vi "Main.vi"() -> ()   [LabVIEW 2013]
uses:
  Type Definitions/3D Model Status.ctl
  Bluetooth/Bluetooth status.ctl
  Type Definitions/Settings File Name.ctl
  <vilib>/Utility/miscctls.llb/LV3DPointTypeDef.ctl
  <vilib>/Instr/_visa.llb/VISA Flush IO Buffer Mask.ctl
  <vilib>/Instr/_visa.llb/VISA Set IO Buffer Mask.ctl
  <vilib>/Utility/xml.llb/Read From XML File(string).vi
  <vilib>/Utility/xml.llb/Write to XML File(string).vi
  <vilib>/picture/3D Picture Control/Object/Create Object (name).vi
  <vilib>/Instr/_visa.llb/VISA Configure Serial Port (Instr).vi
  <vilib>/picture/3D Picture Control/NI_3D Picture Control.lvlib
panel:
  out "Acquire [ms]":u32
  out "Sending [ms]":u32
  in  "VISA resource name":refnum<visa-resource-name>
  in  "Motor 4":u8(slide) scale=0.0..100.0
  in  "Motor 3":u8(slide) scale=0.0..100.0
  in  "Motor 2":u8(slide) scale=0.0..100.0
  in  "Motor 1":u8(slide) scale=0.0..100.0
  out "Press Low":i32 caption="X"
  out "Press High":i32 caption="X"
  out "Temperature":i32
  out "Z Axis":sgl
  out "Zyro 1":i32 caption="X"
  out "Zyro 2":i32 caption="X"
  out "Zyro 3":i32 caption="X"
  out "Zyro 4":i32 caption="X"
  out "Y_Low":i32 caption="Y"
  out "X_Low":i32 caption="X"
  out "Y Axis":sgl
  out "X Axis":sgl
  in  "Stop Bluetooth Button":bool
  in  "Bluetooth Connect Button":bool
  out "Battery":i32
  out "Y_High":i32 caption="Y"
  out "X_High":i32 caption="X"
  out "3D Picture":refnum<vi>(3d-picture)
  in  "Load Model":bool
  in  "Stop Button":bool
  in  "Path to STL File":path=path "C:/Users/Marcin/SkyDrive/Dokumenty/Quadrocopter/LabVIEW 3D Model/Zlozenie.stl"
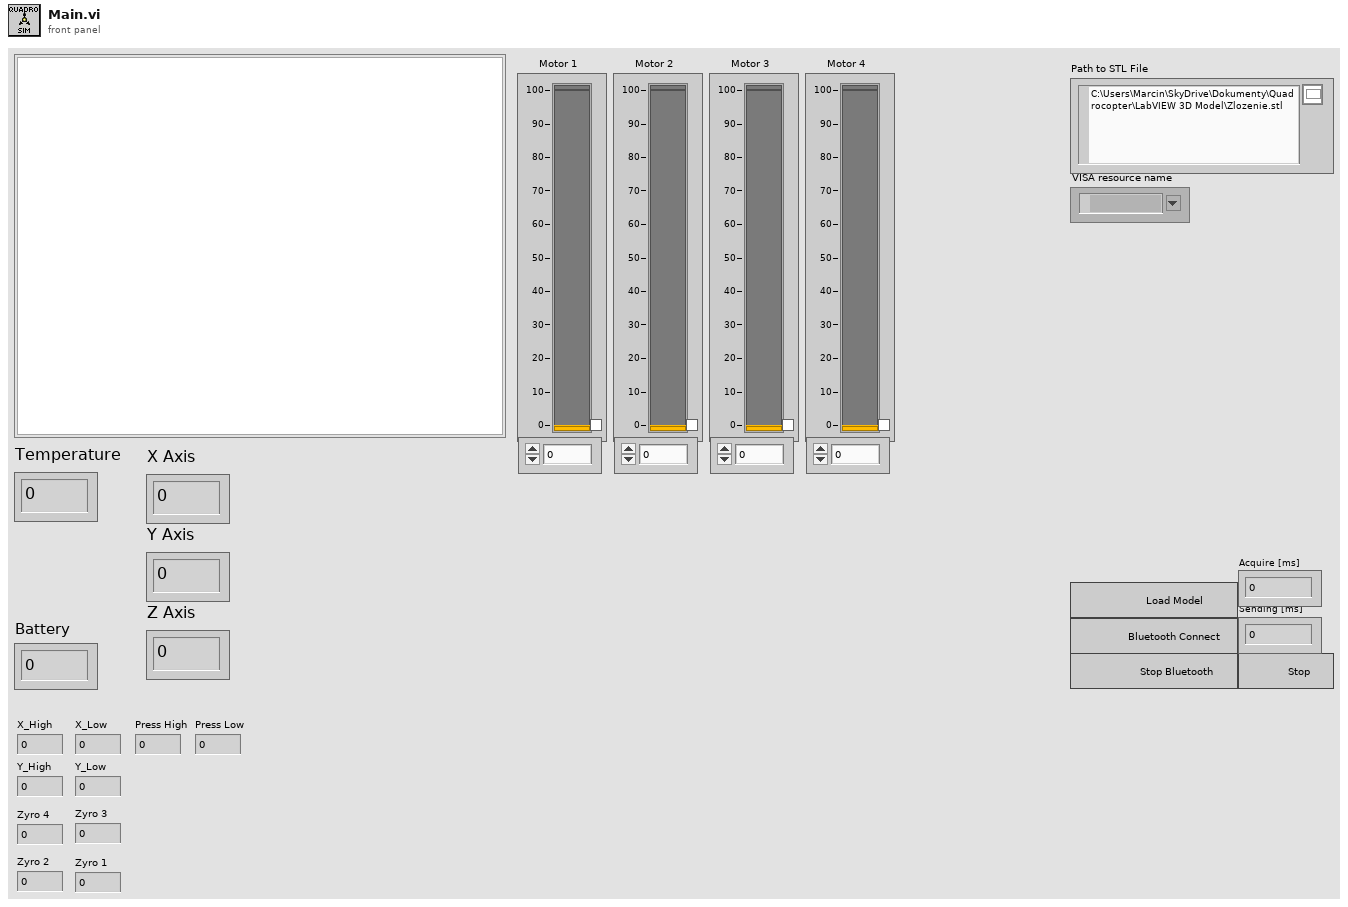
[diagram p1: front panel]
types:
  T1 = typedef "Bluetooth status.ctl" = enum16{"Idle", "Connected"}
  T2 = typedef "3D Model Status.ctl" = enum16{"Idle", "Update"}
  T3 = typedef "VISA Set IO Buffer Mask.ctl" = u16
  T4 = typedef "VISA Flush IO Buffer Mask.ctl" = u16
  T5 = typedef "Settings File Name.ctl" = string
  T6 = typedef "LV3DPointTypeDef.ctl" = cluster{"X":sgl, "Y":sgl, "Z":sgl}
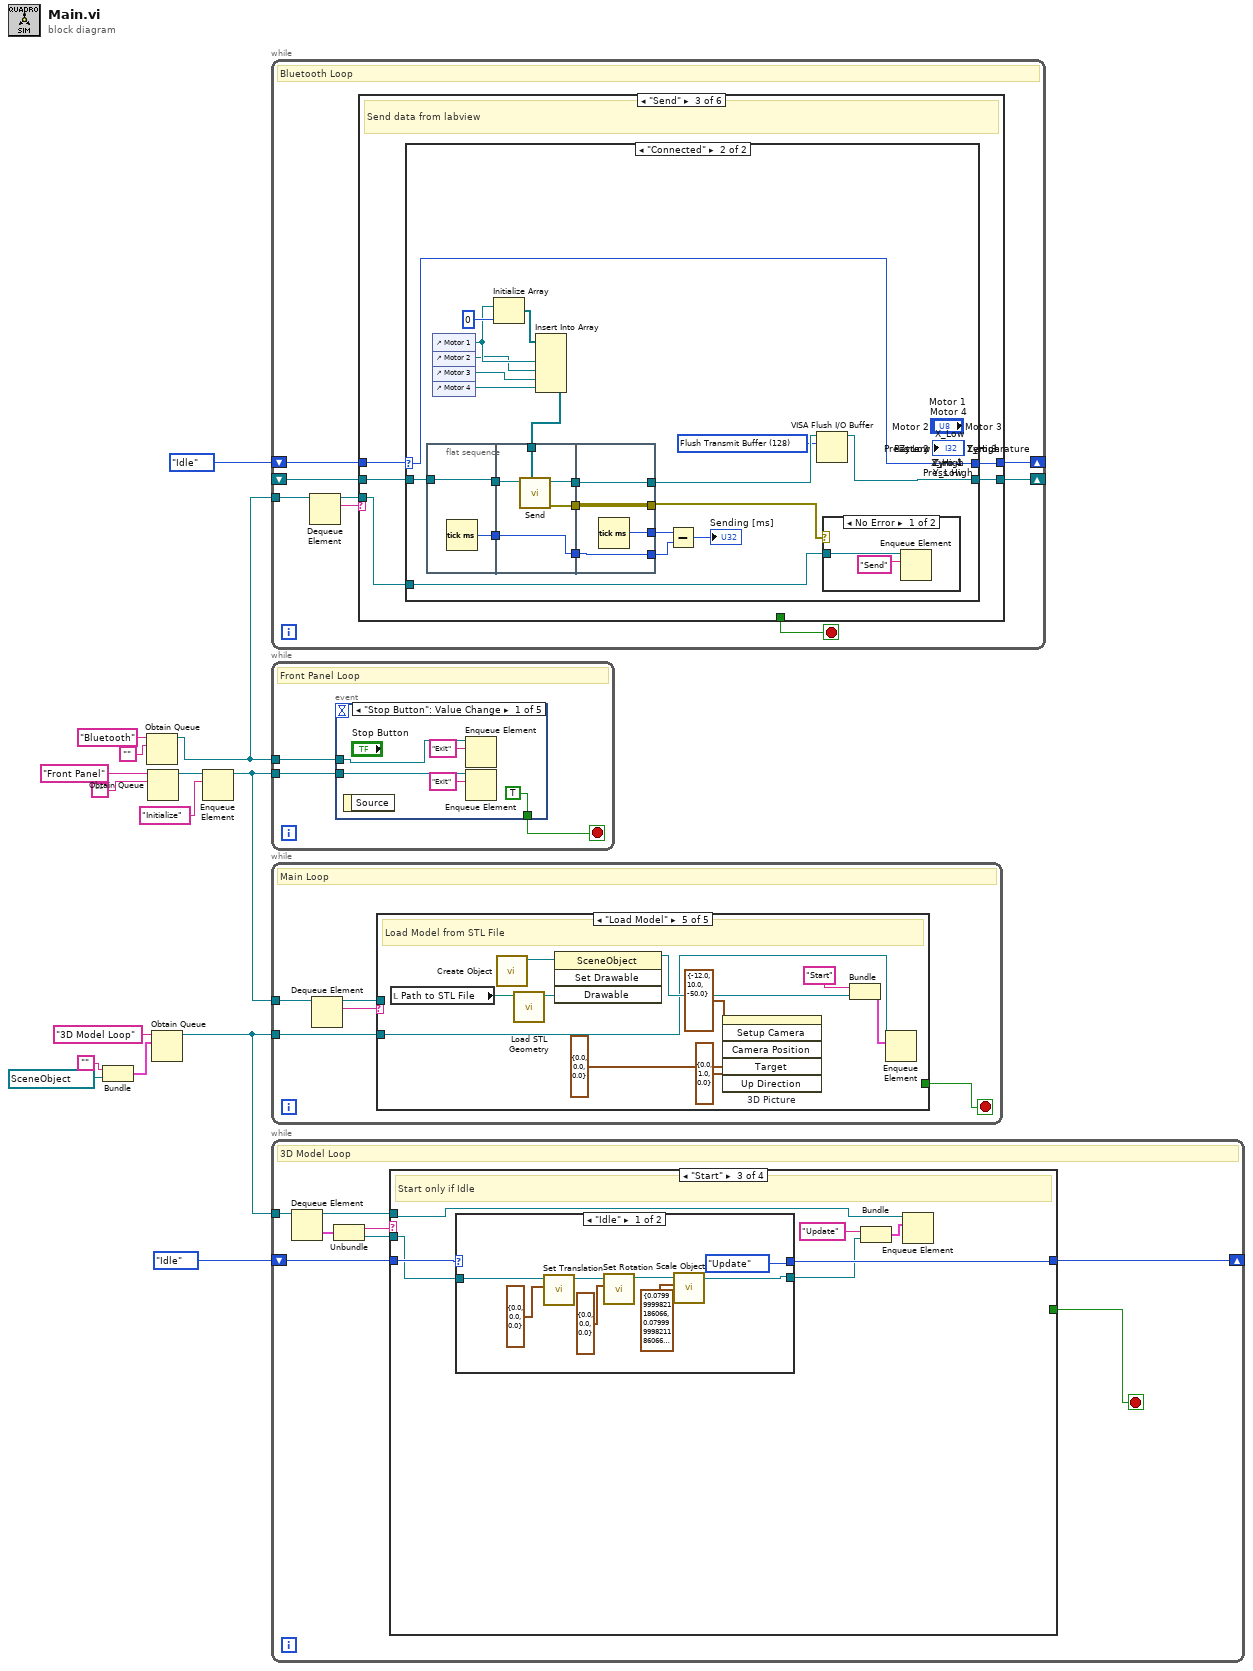
[diagram p0: block diagram]
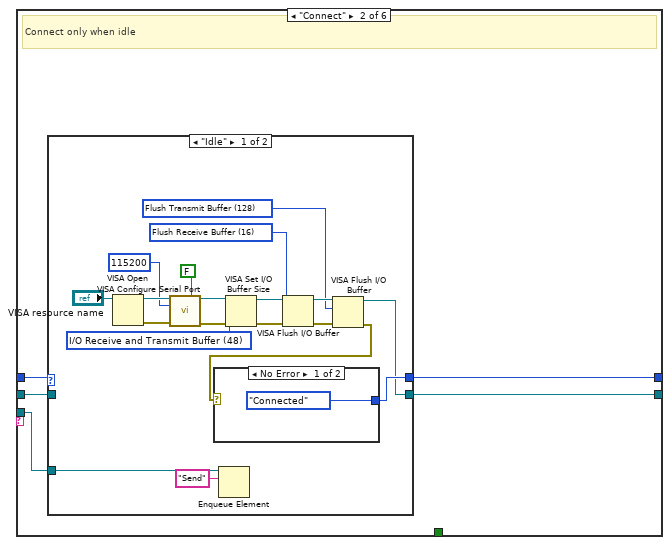
[diagram p3: hidden frame]
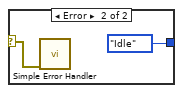
[diagram p4: hidden frame]
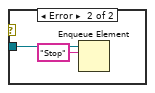
[diagram p7: hidden frame]
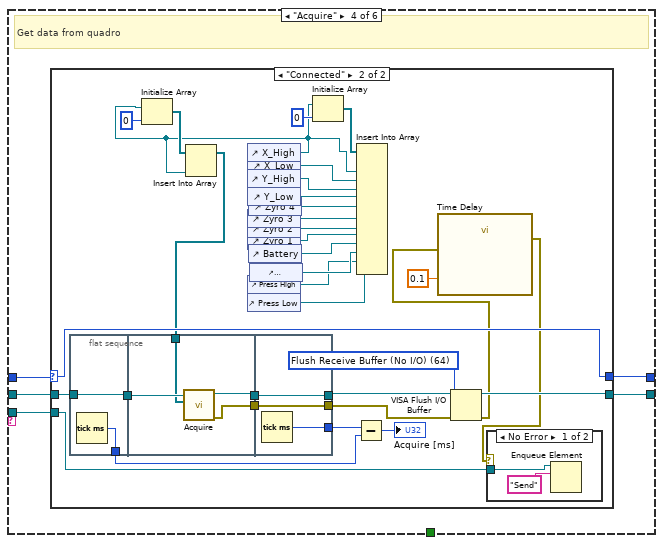
[diagram p8: hidden frame]
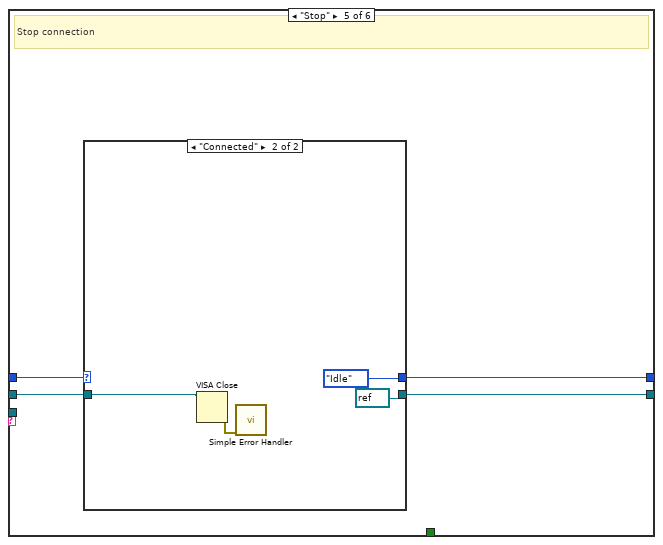
[diagram p11: hidden frame]
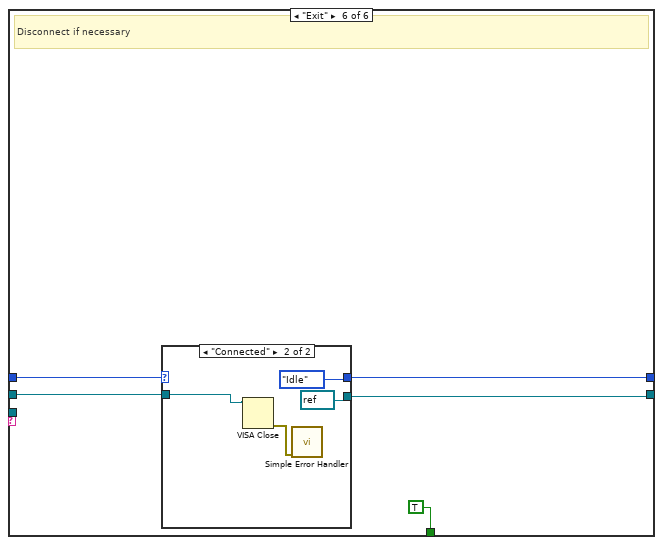
[diagram p13: hidden frame]
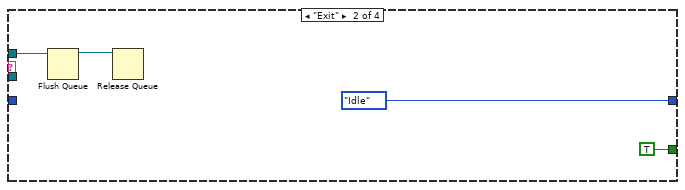
[diagram p16: hidden frame]
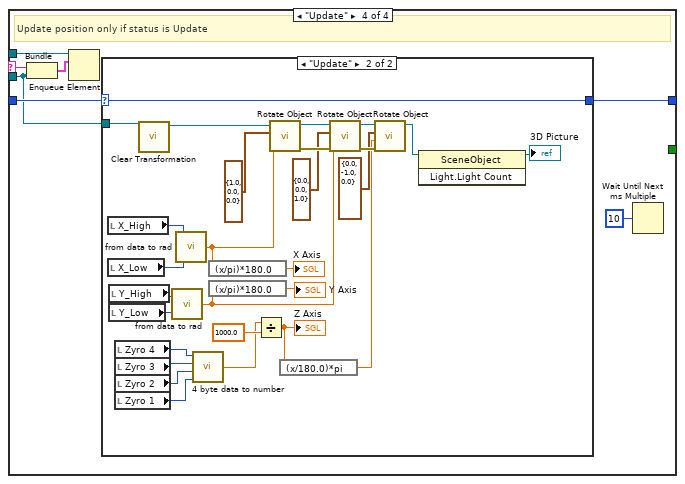
[diagram p18: hidden frame]
diagram:
  n1 = Bundle("", "reference out"=refnum<vi> refnum) -> (w5:cluster{string, "reference out":refnum<vi>})  [unwired: 1 in]
  n2 = Obtain Queue(name (unnamed)="Bluetooth", element data type="") -> (queue out=w2:refnum<queue>)  [unwired: 3 in, 2 out]
  n3 = Obtain Queue(name (unnamed)="Front Panel", element data type="") -> (queue out=w13:refnum<queue>)  [unwired: 3 in, 2 out]
  n4 = Obtain Queue(name (unnamed)="3D Model Loop", element data type=w5) -> (queue out=w9:refnum<queue>)  [unwired: 3 in, 2 out]
  n5 = Enqueue Element(queue=w13, element="Initialize") -> (queue out=w11:refnum<queue>)  [unwired: 2 in, 2 out]
  n6 = while {
    tunnel: w2 -> [w22]
    shift-right: [w19] -> _
    shift-left: Bluetooth_status."Idle" -> [w20]
    shift-right: [w18] -> _
    shift-left: _ -> [w17]
    stop <- w16 stop-if-true
    # "Bluetooth Loop"
    n7 = Dequeue Element(queue=w22) -> (queue out=w21:refnum<queue>, element=w23:string)  [unwired: 2 in, 2 out]
    n8 = case shown="\"Send\"" w23 {
      tunnel: w21 -> [_ w26 w55 w99 _ _]
      tunnel: w20 -> [w24 w30 w59 w103 w153 w163]
      tunnel: [w24 w29 w58 w102 w151 w160] -> w19
      tunnel: [w25 w28 w57 w100 w150 w161] -> w18
      tunnel: w17 -> [w25 w27 w56 w101 w152 w162]
      tunnel: [_ _ _ _ _ TRUE] -> w16
      frame Default {
        # "Do nothing"
      }
      frame "Connect" {
        # "Connect only when idle"
        n9 = case shown="\"Idle\"" w30 {
          selector: w30 -> [_ w53]
          tunnel: [w47 w53] -> w29
          tunnel: [w33 w54] -> w28
          tunnel: w27 -> [_ w54]
          tunnel: w26 -> [w49 _]
          frame "Idle" {
            w31 = T3 48 items=["I/O Receive Buffer"=16, "I/O Transmit Buffer"=32, "I/O Receive and Transmit Buffer"=48] ("Mask")
            w32 = T4 128 items=["Flush Receive Buffer"=16, "Write Transmit Buffer to Device"=32, "Flush Receive Buffer (No I/O)"=64, "Flush Transmit Buffer"=128] ("Mask")
            w37 = T4 16 items=["Flush Receive Buffer"=16, "Write Transmit Buffer to Device"=32, "Flush Receive Buffer (No I/O)"=64, "Flush Transmit Buffer"=128] ("Mask")
            n10 = VISA Open(VISA resource name="VISA resource name") -> (VISA resource name=w46:refnum<visa-resource-name>, error out=w45:errorcluster)  [unwired: 4 in]
            n11 = call-poly "VISA Configure Serial Port"("VISA resource name"=w46, "Enable Termination\nChar (T)"=FALSE ("Enable Termination\nChar (T)"), "baud rate (9600)"=u32 115200, "error in (no error)"=w45) -> ("VISA resource name out"=w43:refnum<visa-resource-name>, "error out"=w44:errorcluster)  [unwired: 10 in]
            n12 = Enqueue Element(queue=w49, element="Send") -> ()  [unwired: 2 in, 3 out]
            n13 = VISA Set I/O Buffer Size(VISA resource name=w43, mask (16)=w31, error in (no error)=w44) -> (VISA resource name out=w41:refnum<visa-resource-name>, error out=w42:errorcluster)  [unwired: 1 in]
            n14 = VISA Flush I/O Buffer(VISA resource name=w41, mask (16)=w37, error in (no error)=w42) -> (VISA resource name out=w35:refnum<visa-resource-name>, error out=w36:errorcluster)
            n15 = VISA Flush I/O Buffer(VISA resource name=w35, mask (16)=w32, error in (no error)=w36) -> (VISA resource name out=w33:refnum<visa-resource-name>, error out=w34:errorcluster)
            n16 = case shown="No Error" w34 {
              selector: w34 -> [_ w52]
              tunnel: [Bluetooth_status."Connected" Bluetooth_status."Idle"] -> w47
              frame No Error {
              }
              frame Error {
                n17 = call <vilib>:"Simple Error Handler.vi"("error in (no error)"=w52) -> ()  [unwired: 4 in, 5 out]
              }
            }
          }
          frame "Connected", Default {
          }
        }
      }
      frame "Send" {
        # "Send data from labview"
        n18 = case shown="\"Connected\"" w59 {
          selector: w59 -> [w61 w66]
          tunnel: [w61 w66] -> w58
          tunnel: [w60 w63] -> w57
          tunnel: w56 -> [w60 w76]
          tunnel: w55 -> [_ w83]
          frame "Idle", Default {
          }
          frame "Connected" {
            w62 = T4 128 items=["Flush Receive Buffer"=16, "Write Transmit Buffer to Device"=32, "Flush Receive Buffer (No I/O)"=64, "Flush Transmit Buffer"=128] ("Mask")
            n19 = flat-sequence {
              tunnel: w76 -> [w85]
              tunnel: [w85] -> w75
              tunnel: [w84] -> w69
              tunnel: w75 -> [w90]
              tunnel: w65 -> [w87]
              tunnel: [w89] -> w73
              tunnel: [w88] -> w72
              tunnel: w69 -> [w86]
              tunnel: [w86] -> w68
              tunnel: [w93] -> w74
              tunnel: [w94] -> w64
              tunnel: w73 -> [w94]
              tunnel: w72 -> [w93]
              tunnel: [w92] -> w71
              tunnel: [w91] -> w70
              tunnel: w68 -> [w91]
              frame #0 {
                n20 = Tick Count (ms)() -> (millisecond timer value=w84:u32)
              }
              frame #1 {
                n21 = call "Send.vi"("Motors input"=w87, "VISA resource name"=w90) -> ("Error Out"=w88:errorcluster, "VISA resource name out"=w89:refnum<visa-resource-name>)  [unwired: 8 in]
              }
              frame #2 {
                n22 = Tick Count (ms)() -> (millisecond timer value=w92:u32)
              }
            }
            n23 = control-ref of="Motor 1"() -> (w80:refnum<vi>)
            n24 = control-ref of="Motor 2"() -> (w79:refnum<vi>)
            n25 = control-ref of="Motor 3"() -> (w78:refnum<vi>)
            n26 = control-ref of="Motor 4"() -> (w77:refnum<vi>)
            n27 = Initialize Array(w80, 0 ("dimension size")) -> (w81:refnum<vi>[])
            n28 = Insert Into Array(array=w81, new element #1=w80, new element #2=w79, new element #3=w78, new element #4=w77) -> (w65:refnum<vi>[])  [unwired: 1 in]
            n29 = Subtract(x=w71, y=w70) -> (x-y=→"Sending [ms]":u32)
            n30 = VISA Flush I/O Buffer(VISA resource name=w64, mask (16)=w62) -> (VISA resource name out=w63:refnum<visa-resource-name>)  [unwired: 1 in, 1 out]
            n31 = case shown="No Error" w74 {
              tunnel: w83 -> [w95 w98]
              frame No Error {
                n32 = Enqueue Element(queue=w95, element="Send") -> ()  [unwired: 2 in, 3 out]
              }
              frame Error {
                n33 = Enqueue Element(queue=w98, element="Stop") -> ()  [unwired: 2 in, 3 out]
              }
            }
          }
        }
      }
      frame "Acquire" {
        # "Get data from quadro"
        n34 = case shown="\"Connected\"" w103 {
          selector: w103 -> [w105 w125]
          tunnel: [w105 w125] -> w102
          tunnel: [w104 w117] -> w100
          tunnel: w101 -> [w104 w120]
          tunnel: w99 -> [_ w115]
          frame "Idle", Default {
          }
          frame "Connected" {
            w116 = T4 64 items=["Flush Receive Buffer"=16, "Write Transmit Buffer to Device"=32, "Flush Receive Buffer (No I/O)"=64, "Flush Transmit Buffer"=128] ("Mask")
            n35 = flat-sequence {
              tunnel: [w142] -> w123
              tunnel: [w141] -> w121
              tunnel: w120 -> [w141]
              tunnel: w121 -> [w146]
              tunnel: [w145] -> w119
              tunnel: [w144] -> w114
              tunnel: w109 -> [w143]
              tunnel: [w149] -> w124
              tunnel: [w148] -> w118
              tunnel: w119 -> [w148]
              tunnel: w114 -> [w147]
              tunnel: [w147] -> w113
              frame #0 {
                n36 = Tick Count (ms)() -> (millisecond timer value=w142:u32)
              }
              frame #1 {
                n37 = call "Acquire.vi"("Controls Ref Array"=w143, "VISA resource name"=w146) -> ("error out"=w144:errorcluster, "VISA resource name out"=w145:refnum<visa-resource-name>)  [unwired: 8 in]
              }
              frame #2 {
                n38 = Tick Count (ms)() -> (millisecond timer value=w149:u32)
              }
            }
            n39 = control-ref of="X_High"() -> (w110:refnum<vi>)
            n40 = Initialize Array(w110, 0 ("dimension size")) -> (w111:refnum<vi>[])
            n41 = Insert Into Array(array=w111, new element=w110) -> (w109:refnum<vi>[])  [unwired: 1 in]
            n42 = control-ref of="X_Low"() -> (w126:refnum<vi>)
            n43 = control-ref of="Y_High"() -> (w137:refnum<vi>)
            n44 = control-ref of="Y_Low"() -> (w138:refnum<vi>)
            n45 = control-ref of="Zyro 3"() -> (w133:refnum<vi>)
            n46 = control-ref of="Zyro 2"() -> (w132:refnum<vi>)
            n47 = control-ref of="Zyro 1"() -> (w131:refnum<vi>)
            n48 = control-ref of="Press High"() -> (w128:refnum<vi>)
            n49 = control-ref of="Press Low"() -> (w127:refnum<vi>)
            n50 = control-ref of="Zyro 4"() -> (w134:refnum<vi>)
            n51 = control-ref of="Battery"() -> (w130:refnum<vi>)
            n52 = control-ref of="Temperature"() -> (w129:refnum<vi>)
            n53 = Initialize Array(w110, 0 ("dimension size")) -> (w136:refnum<vi>[])
            n54 = Subtract(x=w124, y=w123) -> (x-y=→"Acquire [ms]":u32)
            n55 = Insert Into Array(array=w136, new element #1=w110, new element #2=w126, new element #3=w137, new element #4=w138, new element #5=w134, new element #6=w133, new element #7=w132, new element #8=w131, new element #9=w130, new element #10=w129, new element #11=w128, new element #12=w127) -> ()  [unwired: 1 in, 1 out]
            n56 = VISA Flush I/O Buffer(VISA resource name=w118, mask (16)=w116, error in (no error)=w113) -> (VISA resource name out=w117:refnum<visa-resource-name>, error out=w107:errorcluster)
            n57 = call "Time Delay"("error in (no error)"=w107, "Delay Time (s)"=0.1) -> ("error out"=w106:errorcluster)  [unwired: 9 in]
            n58 = case shown="No Error" w106 {
              tunnel: w115 -> [w140 _]
              frame No Error {
                n59 = Enqueue Element(queue=w140, element="Send") -> ()  [unwired: 2 in, 3 out]
              }
              frame Error {
              }
            }
          }
        }
      }
      frame "Stop" {
        # "Stop connection"
        n60 = case shown="\"Connected\"" w153 {
          selector: w153 -> [w155 _]
          tunnel: w152 -> [w154 w157]
          tunnel: [w155 Bluetooth_status."Idle"] -> w151
          tunnel: [w154 refnum<visa-resource-name> refnum ("VISA resource name out")] -> w150
          frame "Idle", Default {
          }
          frame "Connected" {
            n61 = VISA Close(VISA resource name=w157) -> (error out=w158:errorcluster)  [unwired: 1 in]
            n62 = call <vilib>:"Simple Error Handler.vi"("error in (no error)"=w158) -> ()  [unwired: 4 in, 5 out]
          }
        }
      }
      frame "Exit" {
        # "Disconnect if necessary"
        n63 = case shown="\"Connected\"" w163 {
          selector: w163 -> [w165 _]
          tunnel: w162 -> [w166 w169]
          tunnel: [w166 refnum<visa-resource-name> refnum ("VISA resource name out")] -> w161
          tunnel: [w165 Bluetooth_status."Idle"] -> w160
          frame "Idle", Default {
          }
          frame "Connected" {
            n64 = VISA Close(VISA resource name=w169) -> (error out=w167:errorcluster)  [unwired: 1 in]
            n65 = call <vilib>:"Simple Error Handler.vi"("error in (no error)"=w167) -> ()  [unwired: 4 in, 5 out]
          }
        }
      }
    }
  }
  n66 = while {
    tunnel: w11 -> [w173]
    tunnel: w2 -> [w171]
    stop <- w172 stop-if-true
    # "Front Panel Loop"
    n67 = event shown="[0] \"Stop Button\": Value Change" {
      selector: _ -> [_ _ _ _ _]
      dyn-events: _ -> [_ _ _ _ _]
      timeout: _ -> [_ _ _ _ _]
      tunnel: w173 -> [w178 w180 _ _ w186]
      tunnel: [TRUE _ _ _ _] -> w172
      tunnel: w171 -> [w175 _ w182 w184 _]
      event "Stop Button": Value Change {
        n68 = event-data() -> ()  [unwired: 1 in, 1 out]
        n69 = Enqueue Element(queue=w175, element="Exit") -> ()  [unwired: 2 in, 3 out]
        n70 = Enqueue Element(queue=w178, element="Exit") -> ()  [unwired: 2 in, 3 out]
      }
      event "Load Model": Value Change {
        n71 = event-data() -> ()  [unwired: 1 in, 1 out]
        n72 = Enqueue Element(queue=w180, element="Load Model") -> ()  [unwired: 2 in, 3 out]
      }
      event "Bluetooth Connect Button": Value Change {
        n73 = event-data() -> ()  [unwired: 1 in, 1 out]
        n74 = Enqueue Element(queue=w182, element="Connect") -> ()  [unwired: 2 in, 3 out]
      }
      event "Stop Bluetooth Button": Value Change {
        n75 = event-data() -> ()  [unwired: 1 in, 1 out]
        n76 = Enqueue Element(queue=w184, element="Stop") -> ()  [unwired: 2 in, 3 out]
      }
      event "Path to STL File": Value Change {
        n77 = event-data() -> ()  [unwired: 1 in, 1 out]
        n78 = Enqueue Element(queue=w186, element="Save Settings") -> ()  [unwired: 2 in, 3 out]
      }
    }
  }
  n79 = while {
    tunnel: w11 -> [w191]
    tunnel: w9 -> [w187]
    stop <- w189 stop-if-true
    # "Main Loop"
    n80 = Dequeue Element(queue=w191) -> (queue out=w188:refnum<queue>, element=w190:string)  [unwired: 2 in, 2 out]
    n81 = case shown="\"Load Model\"" w190 {
      tunnel: [_ TRUE _ _ _] -> w189
      tunnel: w188 -> [_ w195 _ _ _]
      tunnel: w187 -> [_ w193 _ _ w213]
      frame Default {
      }
      frame "Exit" {
        n82 = Flush Queue(queue=w195) -> (queue out=w194:refnum<queue>)  [unwired: 1 in, 2 out]
        n83 = Release Queue(queue=w194) -> ()  [unwired: 2 in, 3 out]
        n84 = Enqueue Element(queue=w193, element=cluster{string, "reference out":refnum<vi>} {"Exit", "reference out"=refnum}) -> ()  [unwired: 2 in, 3 out]
      }
      frame "Initialize" {
        # "Read settings from XML File, clear 3D Picture"
        n85 = call <vilib>:"Application Directory.vi"() -> ("Application Directory"=w204:path)
        n86 = Build Path(base path=w204, name or relative path=T5 "3D Settings.xml") -> (appended path=w202:path)
        n87 = call-poly <vilib>:"Read From XML File.vi"("XML File Path"=w202) -> ("error out"=w201:errorcluster, "XML Elements"=w200:string)  [unwired: 8 in, 1 out]
        n88 = Unflatten From XML(xml string=w200, type=path "", error in (no error)=w201) -> (value=w198:path)  [unwired: 1 out]
        n89 = local write "Path to STL File"(w198) -> ()
        n90 = local write "3D Picture"(refnum<vi> refnum ("3D Picture")) -> ()
      }
      frame "Save Settings" {
        # "Save settings to XML File"
        n91 = local read "Path to STL File"() -> (w205:path)
        n92 = call <vilib>:"Application Directory.vi"() -> ("Application Directory"=w208:path)
        n93 = Build Path(base path=w208, name or relative path=T5 "3D Settings.xml") -> (appended path=w206:path)
        n94 = Flatten To XML(anything=w205) -> (xml string=w209:string)
        n95 = call-poly <vilib>:"Write to XML File.vi"("XML Input"=w209, "XML File Path"=w206) -> ()  [unwired: 7 in, 3 out]
      }
      frame "Load Model" {
        # "Load Model from STL File"
        n96 = local read "Path to STL File"() -> (w219:path)
        n97 = call-poly <vilib>:"Create Object.vi"() -> ("Scene:New Object"=w218:refnum<vi>)  [unwired: 10 in, 1 out]
        n98 = call <vilib>:"Load STL Geometry.vi"("Model File"=w219) -> ("New Mesh Refnum"=w217:refnum<vi>)  [unwired: 9 in, 1 out]
        n99 = invoke class="SceneObject" method="Set Drawable"(reference=w218, "Drawable"=w217) -> (reference out=w215:refnum<vi>)  [unwired: 2 in, 3 out]
        n100 = invoke on="3D Picture" class="SceneGraphDisp (strict)" method="Setup Camera"("Camera Position"=T6 {"X"=-12.0, "Y"=10.0, "Z"=-50.0}, "Target"=T6 {"X"=0.0, "Y"=0.0, "Z"=0.0}, "Up Direction"=T6 {"X"=0.0, "Y"=1.0, "Z"=0.0}) -> ()  [unwired: 3 in, 6 out]
        n101 = Bundle("Start", "Scene:New Object"=w215) -> (w214:cluster{string, "Scene:New Object":refnum<vi>})  [unwired: 1 in]
        n102 = Enqueue Element(queue=w213, element=w214) -> ()  [unwired: 2 in, 3 out]
      }
    }
  }
  n103 = while {
    tunnel: w9 -> [w227]
    shift-right: [w221] -> _
    shift-left: 3D_Model_Status."Idle" -> [w220]
    stop <- w226 stop-if-true
    # "3D Model Loop"
    n104 = Dequeue Element(queue=w227) -> (queue out=w222:refnum<queue>, element=w225:cluster{string, "reference out":refnum<vi>})  [unwired: 2 in, 2 out]
    n105 = Unbundle(w225) -> (w224:string, "reference out"=w223:refnum<vi>)
    n106 = case shown="\"Start\"" w224 {
      selector: w224 -> [_ _ _ w253]
      tunnel: [_ TRUE _ _] -> w226
      tunnel: w223 -> [_ _ w237 w252]
      tunnel: w222 -> [_ w231 w233 w254]
      tunnel: [w228 3D_Model_Status."Idle" w238 w255] -> w221
      tunnel: w220 -> [w228 _ w239 w256]
      frame Default {
      }
      frame "Exit" {
        n107 = Flush Queue(queue=w231) -> (queue out=w230:refnum<queue>)  [unwired: 1 in, 2 out]
        n108 = Release Queue(queue=w230) -> ()  [unwired: 2 in, 3 out]
      }
      frame "Start" {
        # "Start only if Idle"
        n109 = case shown="\"Idle\"" w239 {
          selector: w239 -> [_ w249]
          tunnel: [3D_Model_Status."Update" w249] -> w238
          tunnel: w237 -> [w244 w248]
          tunnel: [w241 w248] -> w235
          frame "Idle" {
            n110 = call <vilib>:"Set Translation.vi"("Translation"=cluster{"X":sgl, "Y":sgl, "Z":sgl} {"X"=0.0, "Y"=0.0, "Z"=0.0}, "Scene Object"=w244) -> ("Translated Object"=w243:refnum<vi>)  [unwired: 8 in, 1 out]
            n111 = call <vilib>:"Set Rotation.vi"("Axis"=cluster{"X":sgl, "Y":sgl, "Z":sgl} {"X"=0.0, "Y"=0.0, "Z"=0.0}, "Scene Object"=w243) -> ("Rotated Scene Object"=w242:refnum<vi>)  [unwired: 8 in, 1 out]
            n112 = call <vilib>:"Scale Object.vi"("Scale"=cluster{"X":sgl, "Y":sgl, "Z":sgl} {"X"=0.08, "Y"=0.08, "Z"=0.08}, "Scene.Object In"=w242) -> ("Scene.Object Out"=w241:refnum<vi>)  [unwired: 8 in, 1 out]
          }
          frame Default {
            # "Ignore if not idle"
          }
        }
        n113 = Bundle("Update", "reference out"=w235) -> (w234:cluster{string, "reference out":refnum<vi>})  [unwired: 1 in]
        n114 = Enqueue Element(queue=w233, element=w234) -> ()  [unwired: 2 in, 3 out]
      }
      frame "Update" {
        # "Update position only if status is Update"
        n115 = Bundle(w253, "reference out"=w252) -> (w251:cluster{string, "reference out":refnum<vi>})  [unwired: 1 in]
        n116 = Enqueue Element(queue=w254, element=w251) -> ()  [unwired: 2 in, 3 out]
        n117 = case shown="\"Update\"" w256 {
          selector: w256 -> [w257 w285]
          tunnel: [w257 w285] -> w255
          tunnel: w252 -> [_ w284]
          frame Default {
          }
          frame "Update" {
            n118 = local read "X_High"() -> (w273:i32)
            n119 = local read "X_Low"() -> (w272:i32)
            n120 = local read "Y_High"() -> (w271:i32)
            n121 = local read "Y_Low"() -> (w270:i32)
            n122 = local read "Zyro 4"() -> (w266:i32)
            n123 = local read "Zyro 3"() -> (w267:i32)
            n124 = local read "Zyro 2"() -> (w268:i32)
            n125 = local read "Zyro 1"() -> (w269:i32)
            n126 = call <vilib>:"Clear Transformation.vi"("Object Refnum In"=w284) -> ("Object Refnum Out"=w274:refnum<vi>)  [unwired: 9 in, 1 out]
            n127 = call "from data to rad.vi"("Radians low in"=w270, "Radians high in"=w271) -> ("Radians"=w277:sgl)
            n128 = call "from data to rad.vi"("Radians low in"=w272, "Radians high in"=w273) -> ("Radians"=w278:sgl)
            n129 = call "4 byte data to number.vi"("4"=w266, "3"=w267, "2"=w268, "1"=w269) -> ("data out"=w260:dbl)  [unwired: 1 in]
            n130 = expression code="(x/pi)*180.0" ("radians to degrees")(w278) -> (→"X Axis":sgl)
            n131 = expression code="(x/pi)*180.0" ("radians to degrees")(w277) -> (→"Y Axis":sgl)
            n132 = Divide(x=w260, y=1000.0) -> (x/y=w258:dbl)
            "Z Axis" <- w258
            n133 = call <vilib>:"Rotate Object.vi"("Angle"=w278, "Axis"=cluster{"X":sgl, "Y":sgl, "Z":sgl} {"X"=1.0, "Y"=0.0, "Z"=0.0}, "Scene.Object In"=w274) -> ("error out"=w282:errorcluster, "Scene.Object Out"=w281:refnum<vi>)  [unwired: 1 in, 6 out]
            n134 = expression code="(x/180.0)*pi" ("degrees to radians")(w258) -> (w259:dbl)
            n135 = call <vilib>:"Rotate Object.vi"("error in (no error)"=w282, "Angle"=w277, "Axis"=cluster{"X":sgl, "Y":sgl, "Z":sgl} {"X"=0.0, "Y"=0.0, "Z"=1.0}, "Scene.Object In"=w281) -> ("error out"=w264:errorcluster, "Scene.Object Out"=w263:refnum<vi>)  [unwired: 6 out]
            n136 = call <vilib>:"Rotate Object.vi"("error in (no error)"=w264, "Angle"=w259, "Axis"=cluster{"X":sgl, "Y":sgl, "Z":sgl} {"X"=0.0, "Y"=-1.0, "Z"=0.0}, "Scene.Object In"=w263) -> ("Scene.Object Out"=w262:refnum<vi>)  [unwired: 7 out]
            n137 = invoke class="SceneObject" method="Light.Light Count"(reference=w262) -> (reference out=→"3D Picture":refnum<vi>)  [unwired: 2 in, 2 out]
          }
        }
        n138 = Wait Until Next ms Multiple(millisecond multiple=u32 10) -> ()  [unwired: 1 out]
      }
    }
  }
